vi "Select_a_Channel.vi"(6 "Mode":T1(ring), 7 "Extra channel names":string[](array[string]), 8 "Data Files":path[](array[path])) -> (0 "Current Values":string[](array[string]), 1 "Channel Values":string[](array[string]), 2 "Selected Channel Names":string[](array[string]))   [LabVIEW 2020]
uses:
  ADAM Client/Sub VIs/ADAM Controls/Channel_names.ctl
  Data_File_Type.ctl
  ADAM Client/Sub VIs/ADAM Controls/Calib_type_ADAM.ctl
  Globals/Constants_global.vi
panel:
  in  "Tolerance":dbl=1.0 format="%.4f"
  in  "OK":bool
  in  "Search String":string
  in  "Listbox":i32[](listbox)
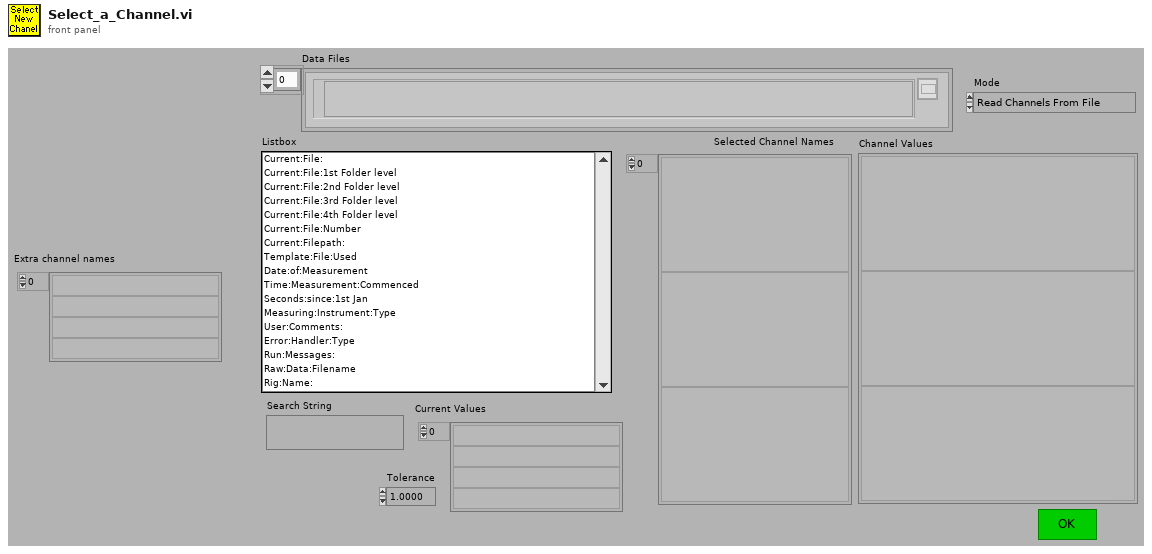
[diagram p1: front panel]
types:
  T1 = enum16{"Read Channels From File", "Read Channels from Server"}
  T2 = typedef "Channel_names.ctl" = enum16{"Active Only", "Active + Off", "All Channels"}
  T3 = typedef "Data_File_Type.ctl" = enum16{"Read All File Types", "Results Files Only", "Raw Data Files Only", "Calibration Files Only", "Gas Desk Files Only", "Old Results Files Only", "Tabulated Data Files Only"}
  T4 = typedef "Ch_description_ADAM.ctl" = cluster{"Ch Name":string, "Type":T5, "Function":T6, "Ch State":T7, "Calibration type":T8, "A":dbl, "B":dbl, "C":dbl, "D":dbl, "Comments":string, "Address":T9, "String":string, "Duty":u16}
  T5 = typedef "Module_type_ADAM.ctl" = string
  T6 = typedef "Function_ADAM.ctl" = enum16{"Analogue Input", "Digital Input", "Event counter", "Event rate", "Analogue Output", "Digital Output", "Relay Output"}
  T7 = typedef "Channel_State.ctl" = enum16{"On", "Off", "Always On", "Always Off"}
  T8 = typedef "Calib_type_ADAM.ctl" = string
  T9 = typedef "Address.ctl" = cluster{"Main":i32, "Ch.":i32, "Sub":i32, "Port Name":string}
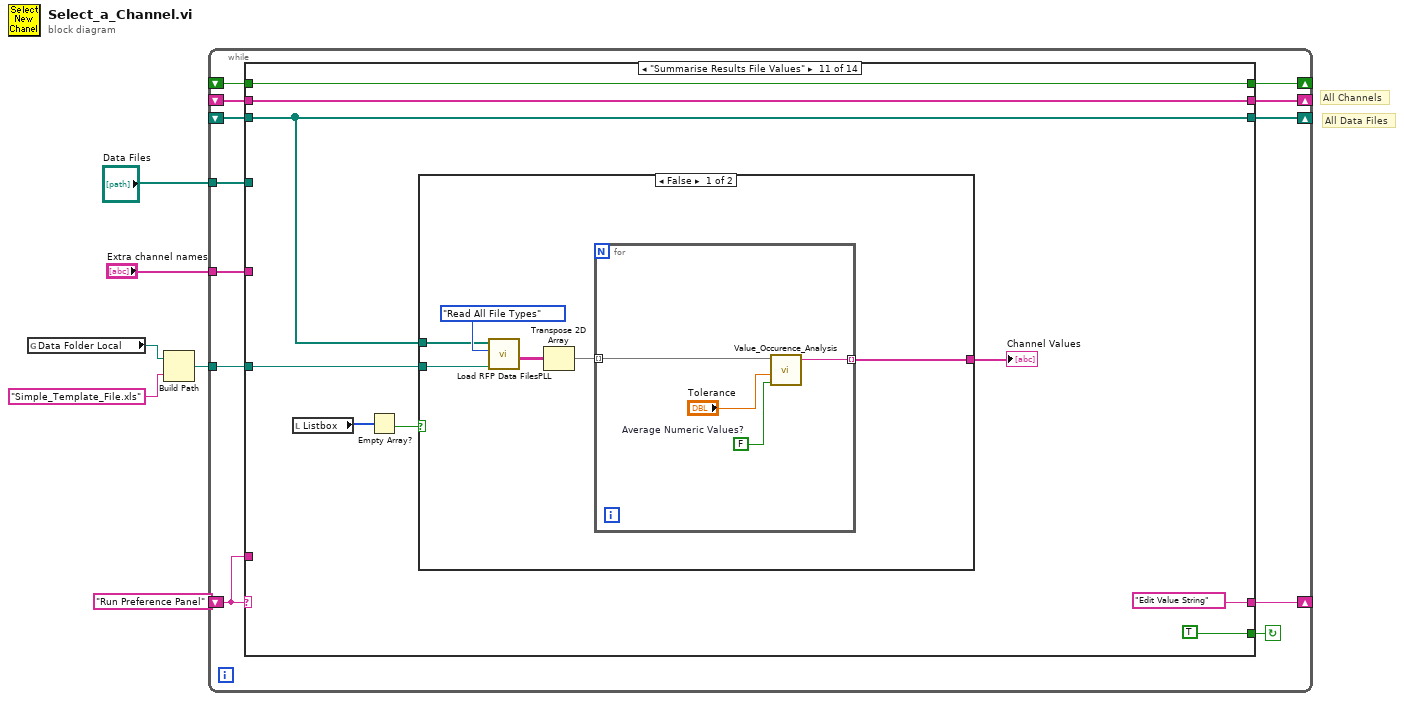
[diagram p0: block diagram]
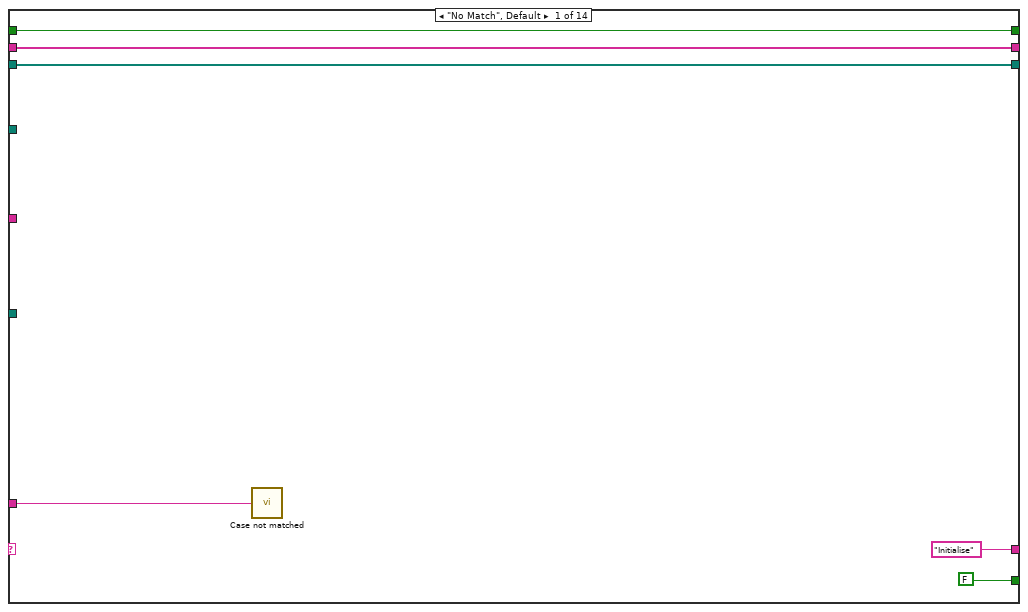
[diagram p2: hidden frame]
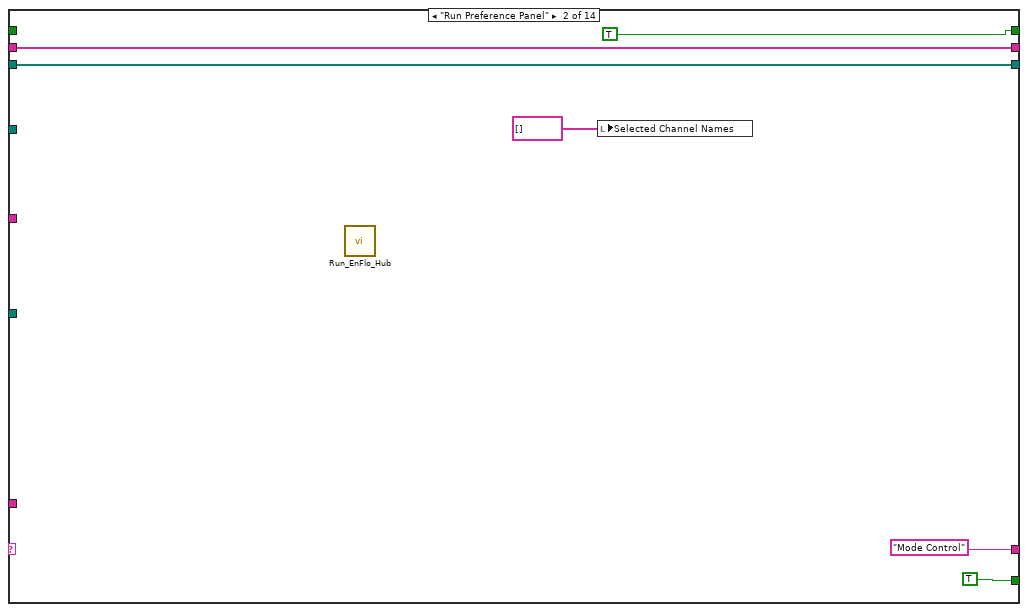
[diagram p3: hidden frame]
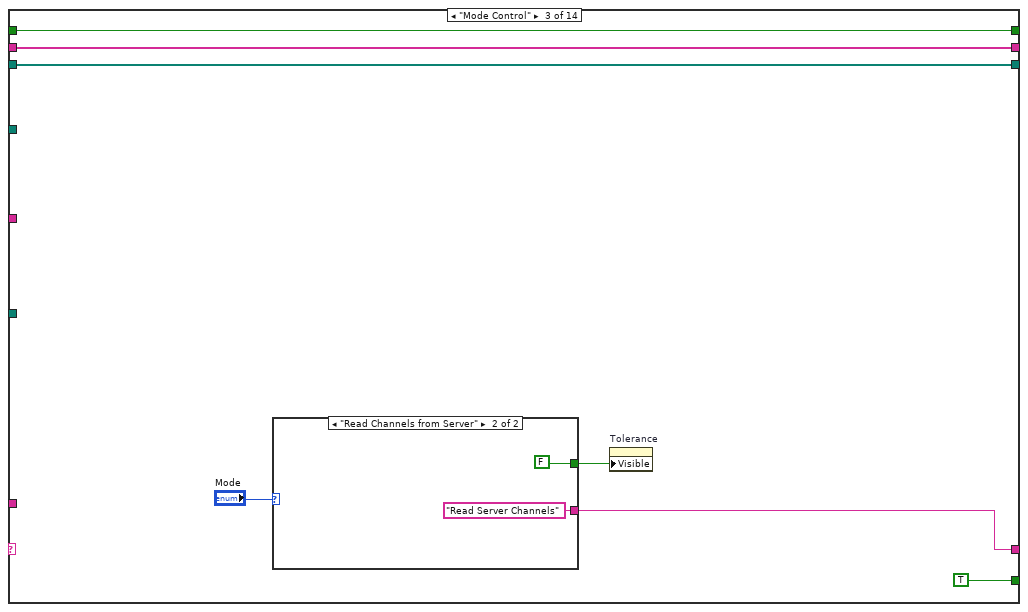
[diagram p4: hidden frame]
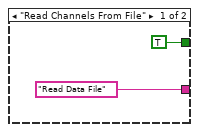
[diagram p5: hidden frame]
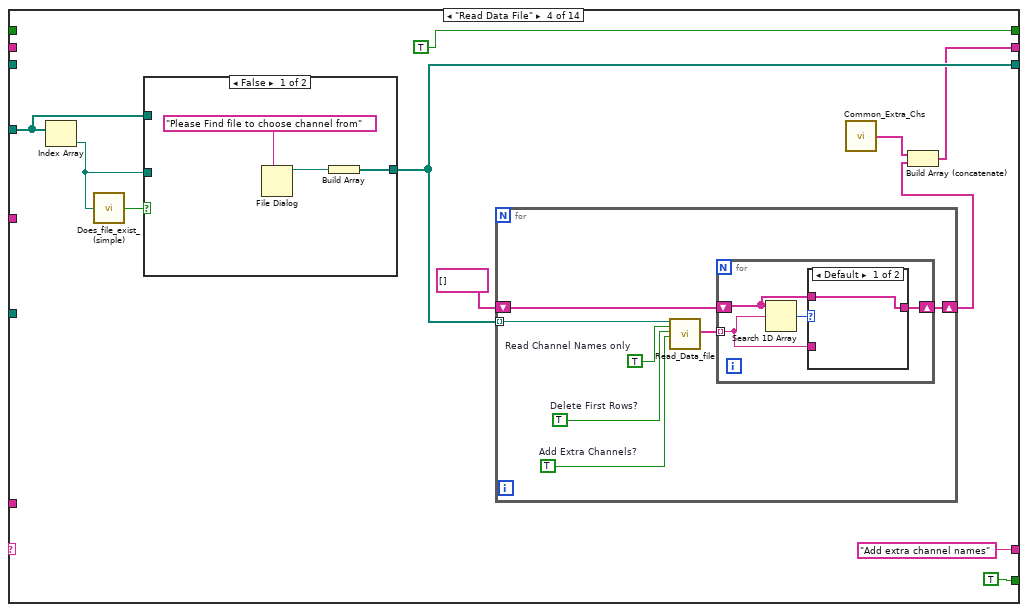
[diagram p6: hidden frame]
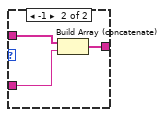
[diagram p7: hidden frame]
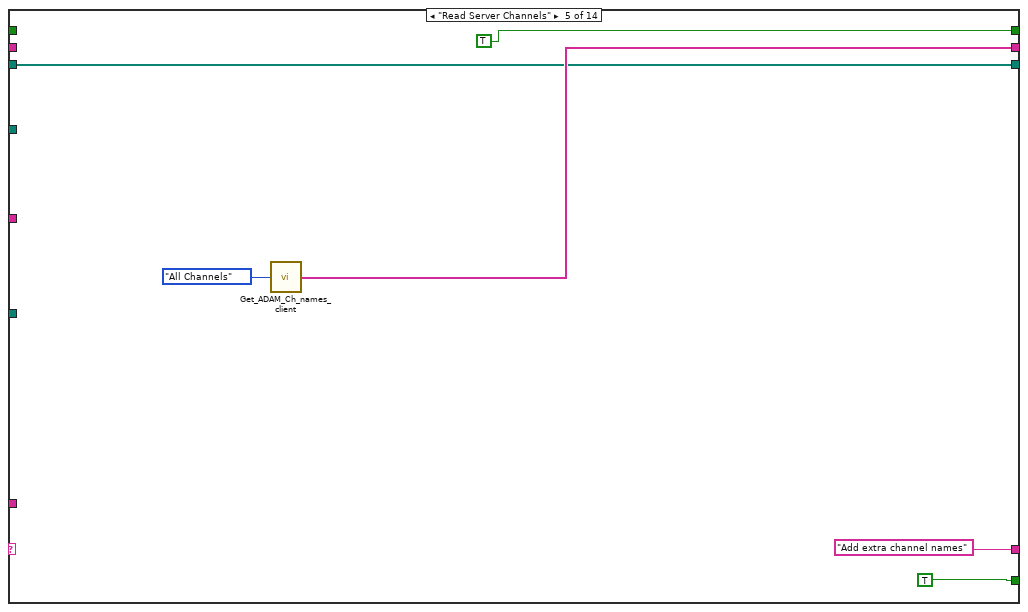
[diagram p9: hidden frame]
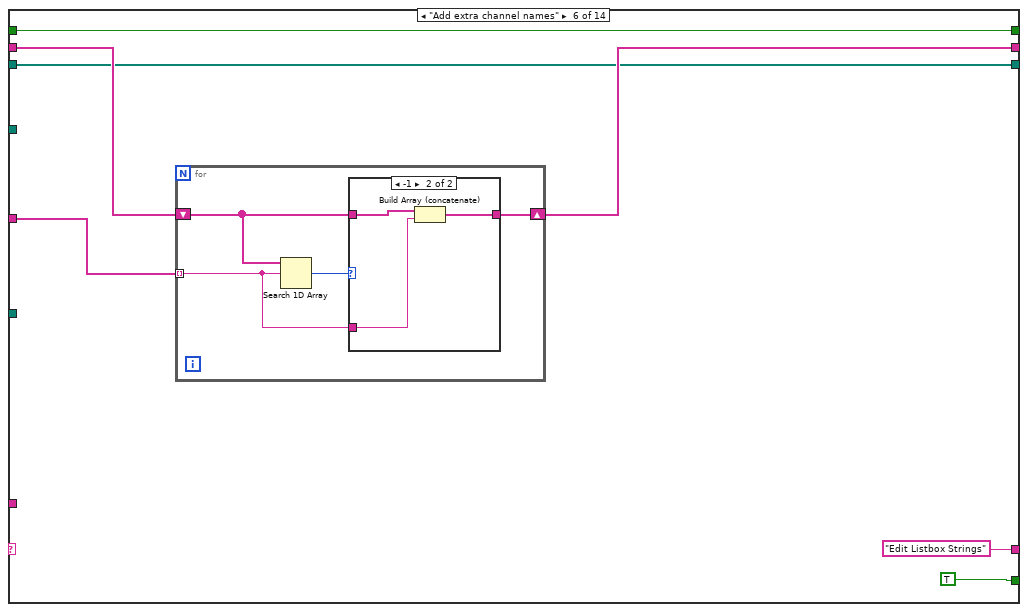
[diagram p10: hidden frame]
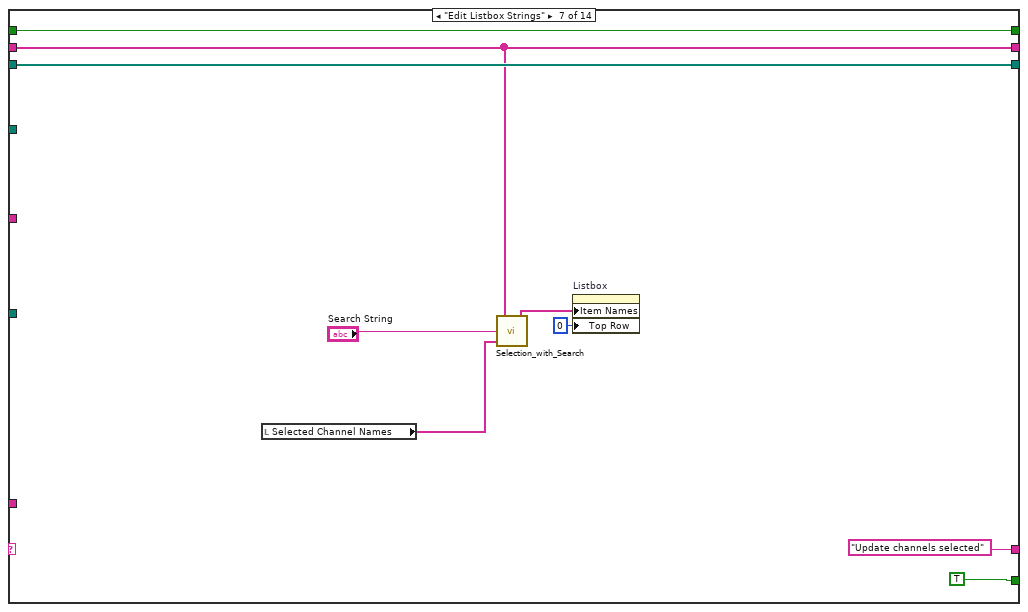
[diagram p12: hidden frame]
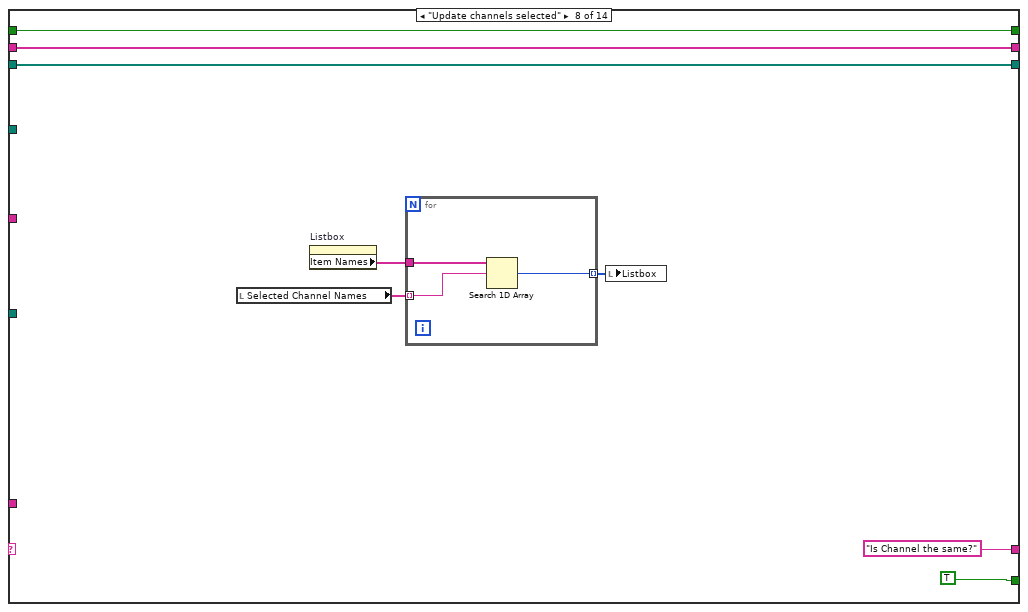
[diagram p13: hidden frame]
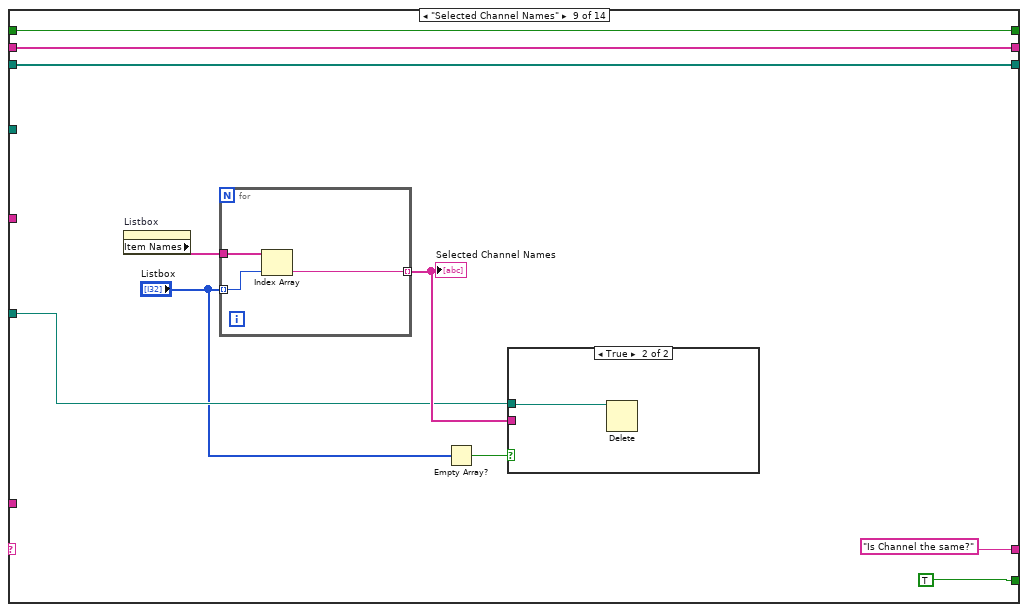
[diagram p14: hidden frame]
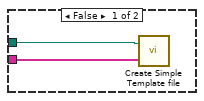
[diagram p15: hidden frame]
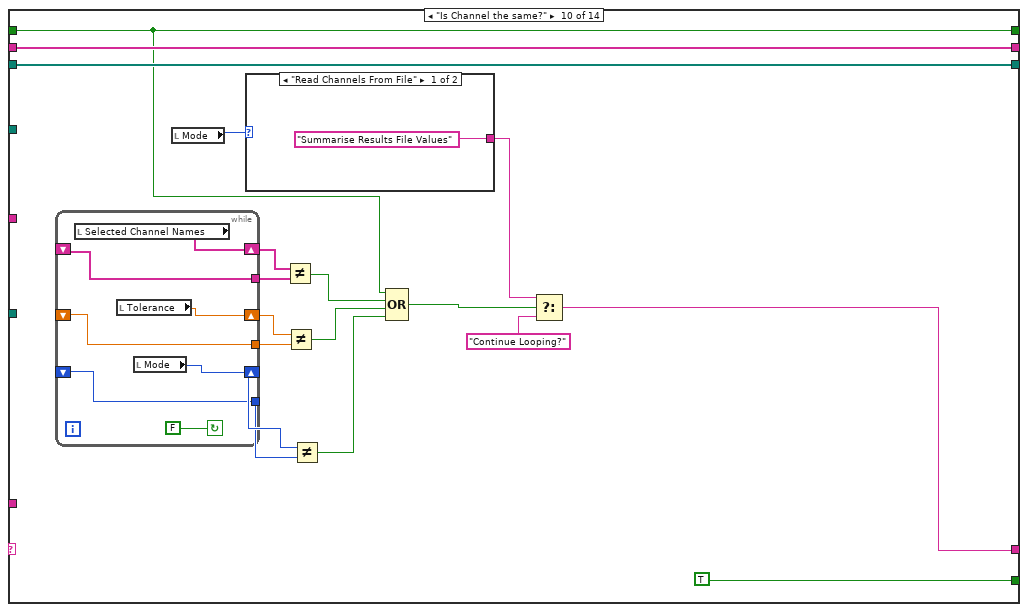
[diagram p16: hidden frame]
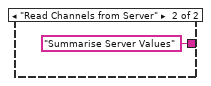
[diagram p17: hidden frame]
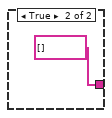
[diagram p18: hidden frame]
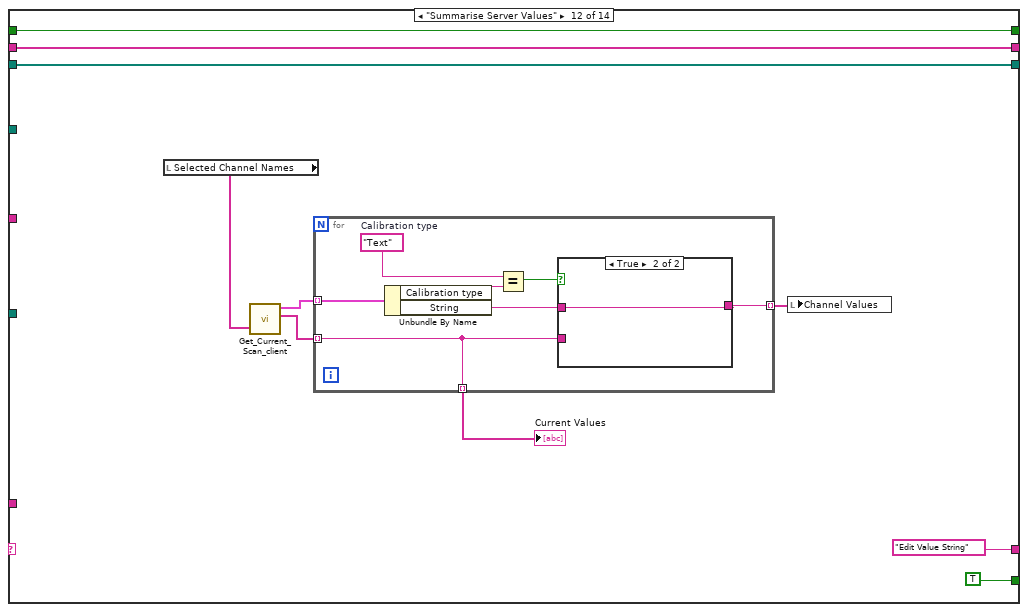
[diagram p19: hidden frame]
diagram:
  # "All Data Files"
  # "All Channels"
  n1 = global read "Constants_global.vi" "Data Folder Local"() -> (w3:path)
  n2 = Build Path(base path=w3, name or relative path="Simple_Template_File.xls") -> (appended path=w1:path)
  n3 = while {
    shift-left: _ -> [w12]
    shift-right: [w14] -> _
    shift-left: _ -> [w13]
    shift-right: [w15] -> _
    shift-left: "Run Preference Panel" -> [w16]
    shift-right: [w17] -> _
    tunnel: "Extra channel names" -> [w11]
    tunnel: "Data Files" -> [w10]
    shift-right: [w8] -> _
    shift-left: _ -> [w9]
    tunnel: w1 -> [w7]
    stop <- w18 continue-if-true
    n4 = case shown="\"Summarise Results File Values\"" w16 {
      tunnel: [FALSE TRUE TRUE TRUE TRUE TRUE TRUE TRUE TRUE TRUE TRUE TRUE TRUE w227] -> w18
      tunnel: ["Initialise" "Mode Control" w34 "Add extra channel names" "Add extra channel names" "Edit Listbox Strings" "Update channels selected" "Is Channel the same?" "Is Channel the same?" w141 "Edit Value String" "Edit Value String" "Continue Looping?" w222] -> w17
      tunnel: w16 -> [w19 _ _ _ _ _ _ _ _ _ _ _ _ _]
      tunnel: [w22 w29 w36 w42 w75 w80 w99 w107 w120 w144 w163 w182 w198 w230] -> w15
      tunnel: [w21 w28 w35 w46 w74 w79 w100 w108 w121 w145 w159 w183 w199 w229] -> w14
      tunnel: w13 -> [w22 w29 w36 _ _ w82 w99 w107 w120 w144 w163 w182 w198 w230]
      tunnel: w12 -> [w21 w28 w35 _ w74 w79 w100 w108 w121 w145 w159 w183 w199 w229]
      tunnel: w11 -> [_ _ _ _ _ w81 _ _ _ _ _ _ _ _]
      tunnel: w10 -> [_ _ _ w48 _ _ _ _ _ _ _ _ _ _]
      tunnel: w9 -> [w20 _ w31 _ _ w78 w93 w102 w117 w129 w161 w176 w195 _]
      tunnel: [w20 TRUE w31 TRUE TRUE w78 w93 w102 w117 w129 w161 w176 w195 FALSE] -> w8
      tunnel: w7 -> [_ _ _ _ _ _ _ _ w115 _ w160 _ _ _]
      frame "No Match", Default {
        n5 = call "Case not matched.vi"("Case Name not Matched"=w19) -> ()
      }
      frame "Run Preference Panel" {
        n6 = call "Run_EnFlo_Hub.vi"() -> ()  [unwired: 1 in, 7 out]
        n7 = local write "Selected Channel Names"(string[] [] ("Selected Channel Names")) -> ()
      }
      frame "Mode Control" {
        n8 = case shown="\"Read Channels from Server\"" "Mode" {
          tunnel: ["Read Data File" "Read Server Channels"] -> w34
          tunnel: [TRUE FALSE] -> w33
          frame "Read Channels From File" {
          }
          frame "Read Channels from Server" {
          }
        }
        n9 = property on="Tolerance" class="DigNum (strict)"("Visible"=w33) -> ()  [unwired: 2 in, 2 out]
      }
      frame "Read Data File" {
        n10 = Index Array(array=w48) -> (element=w49:path)  [unwired: 1 in]
        n11 = call "Does_file_exist_(simple).vi"("Pathname"=w49) -> ("exists?"=w50:bool)
        n12 = case shown="False" w50 {
          tunnel: [w68 w71] -> w46
          tunnel: w49 -> [_ _]
          tunnel: w48 -> [_ w71]
          frame False {
            n13 = File Dialog(7:"Please Find file to choose channel from" ("prompt")) -> (3:w70:path)  [unwired: 1 in, 8 out]
            n14 = Build Array(w70) -> (w68:path[])
          }
          frame True {
          }
        }
        n15 = for {
          tunnel: w46 -> [w59] mode=indexing
          shift-right: [w53] -> w43
          shift-left: string[] [] -> [w54]
          w56 = TRUE  # Read Channel Names only
          w57 = TRUE  # Delete First Rows?
          w58 = TRUE  # Add Extra Channels?
          n16 = call "Read_Data_file.vi"("Results file"=w59, "Read Channel Names only"=w56, "Delete First Rows?"=w57, "Add Extra Channels?"=w58) -> ("Ch names Out"=w55:string[])  [unwired: 3 in, 12 out]
          n17 = for {
            shift-right: [w61] -> w53
            shift-left: w54 -> [w60]
            tunnel: w55 -> [w62] mode=indexing
            n18 = Search 1D Array(1D array=w60, element=w62) -> (index of element=w63:i32)  [unwired: 1 in]
            n19 = case shown="Default" w63 {
              tunnel: w62 -> [_ w67]
              tunnel: [w64 w66] -> w61
              tunnel: w60 -> [w64 w65]
              frame Default {
              }
              frame -1 {
                n20 = Build Array (concatenate)(w65, w67) -> (w66:string[])
              }
            }
          }
        }
        n21 = call "Common_Extra_Chs.vi"() -> ("Common Extra Channels"=w44:string[])
        n22 = Build Array (concatenate)(w44, w43) -> (w42:string[])
      }
      frame "Read Server Channels" {
        n23 = call "Get_ADAM_Ch_names_client.vi"("Channel names set"=Channel_names."All Channels") -> ("Ch names"=w75:string[])
      }
      frame "Add extra channel names" {
        n24 = for {
          shift-right: [w86] -> w80
          shift-left: w82 -> [w87]
          tunnel: w81 -> [w85] mode=indexing
          n25 = Search 1D Array(1D array=w87, element=w85) -> (index of element=w88:i32)  [unwired: 1 out]
          n26 = case shown="-1" w88 {
            tunnel: w87 -> [w89 w92]
            tunnel: [w89 w91] -> w86
            tunnel: w85 -> [_ w90]
            frame 0, Default {
            }
            frame -1 {
              n27 = Build Array (concatenate)(w92, w90) -> (w91:string[])
            }
          }
        }
      }
      frame "Edit Listbox Strings" {
        n28 = local read "Selected Channel Names"() -> (w95:string[])
        n29 = call "Selection_with_Search.vi"("Selected Channel Names"=w95, "Search String"="Search String", "All Channel Names"=w99) -> ("Item Names"=w96:string[])
        n30 = property on="Listbox" class="LstBox (strict)"("Item Names"=w96, "Top Row"=0) -> ()  [unwired: 2 in, 2 out]
      }
      frame "Update channels selected" {
        n31 = local read "Selected Channel Names"() -> (w104:string[])
        n32 = property on="Listbox" class="LstBox (strict)"() -> ("Item Names"=w105:string[])  [unwired: 2 in, 2 out]
        n33 = for {
          tunnel: w105 -> [w112]
          tunnel: w104 -> [w111] mode=indexing
          tunnel: [w110] -> w103 mode=indexing
          n34 = Search 1D Array(1D array=w112, element=w111) -> (index of element=w110:i32)  [unwired: 1 out]
        }
        n35 = local write "Listbox"(w103) -> ()
      }
      frame "Selected Channel Names" {
        n36 = property on="Listbox" class="LstBox (strict)"() -> ("Item Names"=w118:string[])  [unwired: 2 in, 2 out]
        n37 = for {
          tunnel: w118 -> [w128]
          tunnel: "Listbox" -> [w127] mode=indexing
          tunnel: [w126] -> w116 mode=indexing
          n38 = Index Array(array=w128, index=w127) -> (element=w126:string)
        }
        "Selected Channel Names" <- w116
        n39 = Empty Array?(array="Listbox") -> (empty?=w113:bool)
        n40 = case shown="True" w113 {
          tunnel: w116 -> [w124 _]
          tunnel: w115 -> [w123 w125]
          frame False {
            n41 = call "Create Simple Template file.vi"("Wanted Channels"=w124, "Template File"=w123) -> ()  [unwired: 2 in]
          }
          frame True {
            n42 = Delete(path (use dialog)=w125) -> ()  [unwired: 4 in, 3 out]
          }
        }
      }
      frame "Is Channel the same?" {
        n43 = while {
          tunnel: [w149] -> w133
          shift-left: _ -> [w149]
          shift-right: [w148] -> w134
          tunnel: [w150] -> w140
          shift-left: _ -> [w150]
          shift-right: [w151] -> w139
          tunnel: [w152] -> w142
          shift-left: _ -> [w152]
          shift-right: [w153] -> w143
          stop <- FALSE continue-if-true
          n44 = local read "Selected Channel Names"() -> (w153:string[])
          n45 = local read "Tolerance"() -> (w151:dbl)
          n46 = local read "Mode"() -> (w148:T1)
        }
        n47 = local read "Mode"() -> (w135:T1)
        n48 = case shown="\"Read Channels From File\"" w135 {
          tunnel: ["Summarise Results File Values" "Summarise Server Values"] -> w131
          frame "Read Channels From File" {
          }
          frame "Read Channels from Server" {
          }
        }
        n49 = Not Equal?(x=w143, y=w142) -> (x != y?=w138:bool)
        n50 = Not Equal?(x=w139, y=w140) -> (x != y?=w137:bool)
        n51 = Not Equal?(x=w134, y=w133) -> (x != y?=w132:bool)
        n52 = Compound Arithmetic op=OR(w129, w138, w137, w132) -> (w136:bool)
        n53 = Select(t=w131, s=w136, f="Continue Looping?") -> (s? t:f=w141:string)
      }
      frame "Summarise Results File Values" {
        n54 = local read "Listbox"() -> (w156:i32[])
        n55 = Empty Array?(array=w156) -> (empty?=w157:bool)
        n56 = case shown="False" w157 {
          tunnel: w160 -> [w170 _]
          tunnel: w159 -> [w168 _]
          tunnel: [w165 string[] []] -> w158
          frame False {
            n57 = call "Load RFP Data FilesPLL.vi"("Template"=w170, "File Types to Read"=Data_File_Type."Read All File Types", "Files"=w168) -> ("Channel Values Out"=w167:string[][])  [unwired: 5 in, 3 out]
            n58 = Transpose 2D Array(2D array=w167) -> (transposed array=w166:string[][])
            n59 = for {
              tunnel: [w173] -> w165 mode=indexing
              tunnel: w166 -> [w171] mode=indexing
              w172 = FALSE  # Average Numeric Values?
              n60 = call "Value_Occurence_Analysis.vi"("Average Numeric Values?"=w172, "Tolerance"="Tolerance", "String Array"=w171) -> ("Output String"=w173:string)  [unwired: 1 in, 2 out]
            }
          }
          frame True {
          }
        }
        "Channel Values" <- w158
      }
      frame "Summarise Server Values" {
        n61 = local read "Selected Channel Names"() -> (w181:string[])
        n62 = call "Get_Current_Scan_client.vi"("multipleChannels"=w181) -> ("Ch Description Array"=w180:T4[], "String values"=w179:string[])  [unwired: 1 in, 2 out]
        n63 = for {
          tunnel: w180 -> [w188] mode=indexing
          tunnel: w179 -> [w187] mode=indexing
          tunnel: [w189] -> w177 mode=indexing
          tunnel: [w187] -> w178 mode=indexing
          w186 = T8 "Text"  # Calibration type
          n64 = Unbundle By Name(w188) -> ("Calibration type"=w192:T8, "String"=w190:string)
          n65 = Equal?(x=w186, y=w192) -> (x = y?=w191:bool)
          n66 = case shown="True" w191 {
            tunnel: [w193 w194] -> w189
            tunnel: w190 -> [_ w194]
            tunnel: w187 -> [w193 _]
            frame False {
            }
            frame True {
            }
          }
        }
        "Current Values" <- w178
        n67 = local write "Channel Values"(w177) -> ()
      }
      frame "Edit Value String" {
        n68 = local read "Channel Values"() -> (w197:string[])
        n69 = for {
          tunnel: w197 -> [w203] mode=indexing
          tunnel: [w202] -> w196 mode=indexing
          n70 = call "Fast_string_Replace.vi"("Replace match with:"="", "Input String"=w203, "regular expression"="\"") -> ("Output String"=w204:string)  [unwired: 2 out]
          n71 = call "Get_array_values_fr_String.vi"("String Value"=w204) -> ("String array"=w209:string[])  [unwired: 1 out]
          n72 = for {
            shift-right: [w210] -> w202
            shift-left: "" -> [w213]
            tunnel: w209 -> [w212] mode=indexing
            tunnel: "\n" -> [w211]
            n73 = Concatenate Strings(w213, w212, w211) -> (w210:string)
          }
        }
        n74 = local write "Channel Values"(w196) -> ()
      }
      frame "Continue Looping?" {
        n75 = property on="Selected Channel Names" class="Arr (strict)"() -> ("Index Values"=w215:u32[])  [unwired: 2 in, 2 out]
        n76 = while {
          tunnel: [w232] -> w221
          shift-left: _ -> [w232]
          shift-right: [w233] -> w220
          tunnel: [w235] -> w225
          shift-left: _ -> [w235]
          shift-right: [w234] -> w226
          stop <- FALSE continue-if-true
          n77 = local read "Search String"() -> (w233:string)
          n78 = local read "Mode"() -> (w234:T1)
        }
        n79 = property on="Channel Values" class="Arr (strict)"("Index Values"=w215) -> ()  [unwired: 2 in, 2 out]
        n80 = Equal?(x=w226, y=w225) -> (x = y?=w224:bool)
        n81 = Equal?(x=w220, y=w221) -> (x = y?=w219:bool)
        n82 = Select(t="Selected Channel Names", s=w219, f="Edit Listbox Strings") -> (s? t:f=w216:string)
        n83 = Not(x="OK") -> (.not. x?=w227:bool)
        n84 = Select(t=w216, s=w224, f="Mode Control") -> (s? t:f=w222:string)
      }
    }
  }
